vi "Draw Title.vi"(7 "Filters":string[](array[string]), 9 "Background Color":u32(colorbox)=16777215, 10 "Text Color":u32(colorbox), 11 "Title":string="Test Title") -> (3 "new picture":picture)   [LabVIEW 2016, in "MetaDataObj.lvclass"]
uses:
  <resource>/dialog/NewProjectWizard/MetaDataObj/MetaDataObj.lvclass
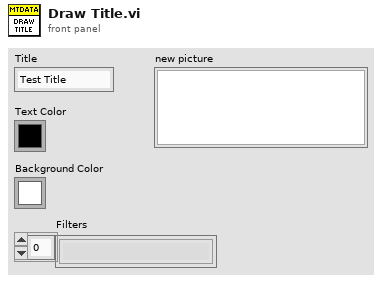
[diagram p1: front panel]
types:
  T1 = cluster{"Font Name:":string, "Size":i16, "Strikeout?":bool, "Italic?":bool, "Underline?":bool, "Outline?":bool, "Shadow?":bool, "Bold?":bool}
  T2 = enum16{"User-specified Font", "Application Font", "System Font", "Dialog Font"}
  T3 = enum32{"invalid OS target", "Mac OS", "Windows 3.1", "Windows 95/NT", "Solaris 1", "Solaris 2", "HP-UX", "PowerMAX", "Linux", "Irix", "Rhapsody", "BeOS", "AIX", "OSF1", "VxWorks", "PharLap", "Carbon", "RTX", "Windows x64", "Linux x64", "Mac OS X x64"}
  T4 = cluster{"left":i16, "top":i16, "right":i16, "bottom":i16}
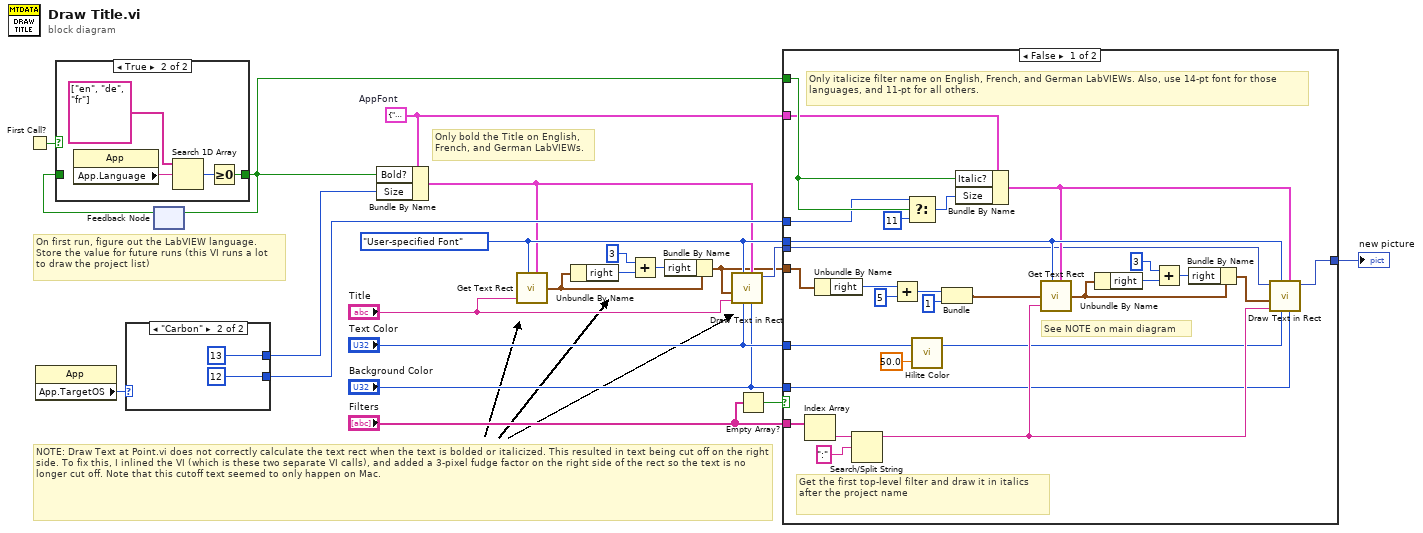
[diagram p0: block diagram]
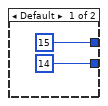
[diagram p2: hidden frame]
diagram:
  w14 = T1 {"Font Name:"="Application Font", "Size"=15, "Strikeout?"=FALSE, "Italic?"=FALSE, "Underline?"=FALSE, "Outline?"=FALSE, "Shadow?"=FALSE, "Bold?"=FALSE}  # AppFont
  w11 = T2."User-specified Font" ("desired font(Application)")
  # "NOTE: Draw Text at Point.vi does not correctly calculate the text rect when the text is bolded or italicized. This resulted in text being cut off on the right side. To fix this, I inlined the VI (which is these two separate VI calls), and added a 3-pixel fudge factor on the right side of the rect so the text is no longer cut off. Note that this cutoff text seemed to only happen on Mac."
  # "On first run, figure out the LabVIEW language.\nStore the value for future runs (this VI runs a lot\nto draw the project list)"
  # "Only bold the Title on English, French, and German LabVIEWs."
  n1 = First Call?() -> (First Call?: T/F=w17:bool)
  n2 = property class="App"() -> ("App.TargetOS"=w15:T3)  [unwired: 2 in, 2 out]
  n3 = case shown="\"Carbon\"" w15 {
    tunnel: [i16 15 ("Size") i16 13 ("Size")] -> w13
    tunnel: [i16 14 ("Size") i16 12 ("Size")] -> w12
    frame Default {
    }
    frame "Carbon" {
    }
  }
  n4 = feedback #1() -> (w18:bool)  [unwired: 1 in]
  n5 = case shown="True" w17 {
    tunnel: [w26 w27] -> w16
    tunnel: w18 -> [w26 _]
    frame False {
    }
    frame True {
      n6 = property class="App"() -> ("App.Language"=w30:string)  [unwired: 2 in, 2 out]
      n7 = Search 1D Array(1D array=string[] ["en", "de", "fr"], element=w30) -> (index of element=w28:i32)  [unwired: 1 in]
      n8 = Greater Or Equal To 0?(x=w28) -> (x >= 0?=w27:bool)
    }
  }
  n9 = feedback-in #1(w16) -> ()
  n10 = Bundle By Name(cluster=w14, "Bold?"=w16, "Size"=w13) -> (w10:T1)
  n11 = call <vilib>:"Get Text Rect.vi"("desired font(Application)"=w11, "text"="Title", "[user-specified font]"=w10) -> ("rect"=w5:T4)  [unwired: 6 in]
  n12 = Unbundle By Name(w5) -> ("right"=w4:i16)
  n13 = Add(x=i16 3, y=w4) -> (x+y=w3:i16)
  n14 = Bundle By Name(cluster=w5, "right"=w3) -> (w1:T4)
  n15 = call <vilib>:"Draw Text in Rect.vi"("BG color(transparent)"="Background Color", "[user-specified font]"=w10, "text color(black)"="Text Color", "desired font(Application)"=w11, "text"="Title", "rect"=w1) -> ("new picture"=w9:picture)  [unwired: 5 in]
  n16 = Empty Array?(array="Filters") -> (empty?=w20:bool)
  n17 = case shown="False" w20 {
    tunnel: w1 -> [w58 _]
    tunnel: w9 -> [w31 w59]
    tunnel: w11 -> [w37 _]
    tunnel: "Text Color" -> [w55 _]
    tunnel: "Background Color" -> [w33 _]
    tunnel: [w38 w59] -> w21
    tunnel: "Filters" -> [w54 _]
    tunnel: w16 -> [w46 _]
    tunnel: w14 -> [w45 _]
    tunnel: w12 -> [w44 _]
    frame False {
      # "See NOTE on main diagram"
      # "Only italicize filter name on English, French, and German LabVIEWs. Also, use 14-pt font for those languages, and 11-pt for all others."
      # "Get the first top-level filter and draw it in italics after the project name"
      n18 = Index Array(array=w54) -> (element=w53:string)  [unwired: 1 in]
      n19 = Unbundle By Name(w58) -> ("right"=w57:i16)
      n20 = Search/Split String(string=w53, search string/char (-)=":") -> (substring before match=w35:string)  [unwired: 1 in, 2 out]
      n21 = Add(x=w57, y=i16 5) -> (x+y=w51:i16)
      n22 = Select(t=w44, s=w46, f=i16 11 ("Size")) -> (s? t:f=w48:i16)
      n23 = call <vilib>:"Hilite Color.vi"("Percentage(30)"=50.0, "Color In"=w55) -> ("Hilite"=w34:u32)  [unwired: 1 out]
      n24 = Bundle(w51, "y"=i16 1) -> (w32:cluster{i16, "y":i16})  [unwired: 1 in]
      n25 = Bundle By Name(cluster=w45, "Italic?"=w46, "Size"=w48) -> (w36:T1)
      n26 = call <vilib>:"Get Text Rect.vi"("desired font(Application)"=w37, "origin(0,0)"=w32, "text"=w35, "[user-specified font]"=w36) -> ("rect"=w39:T4)  [unwired: 5 in]
      n27 = Unbundle By Name(w39) -> ("right"=w40:i16)
      n28 = Add(x=i16 3, y=w40) -> (x+y=w41:i16)
      n29 = Bundle By Name(cluster=w39, "right"=w41) -> (w43:T4)
      n30 = call <vilib>:"Draw Text in Rect.vi"("BG color(transparent)"=w33, "[user-specified font]"=w36, "text color(black)"=w34, "desired font(Application)"=w37, "text"=w35, "rect"=w43, "picture"=w31) -> ("new picture"=w38:picture)  [unwired: 4 in]
    }
    frame True {
      # "No Filter (this should never happen)"
    }
  }
  "new picture" <- w21
